vi "Detector Setup.vi"(8 "error in (no error)":errorcluster, 11 "Detector Class in":refnum<class "Detector Class.lvclass">) -> (0 "error out":errorcluster, 2 "Detector Config.Detector":u16, 3 "Detector Class out":refnum<class "Detector Class.lvclass">)   [LabVIEW 2021, in "Detector Class.lvclass"]
uses:
  Detector Class.lvclass
  Detector Class.lvclass/Detector Class.ctl
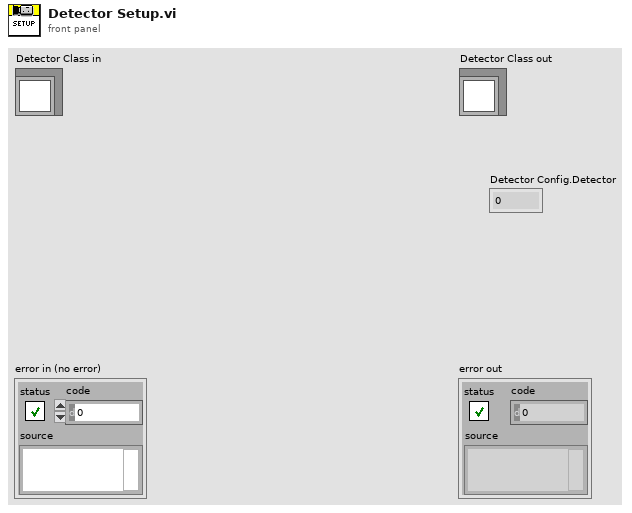
[diagram p1: front panel]
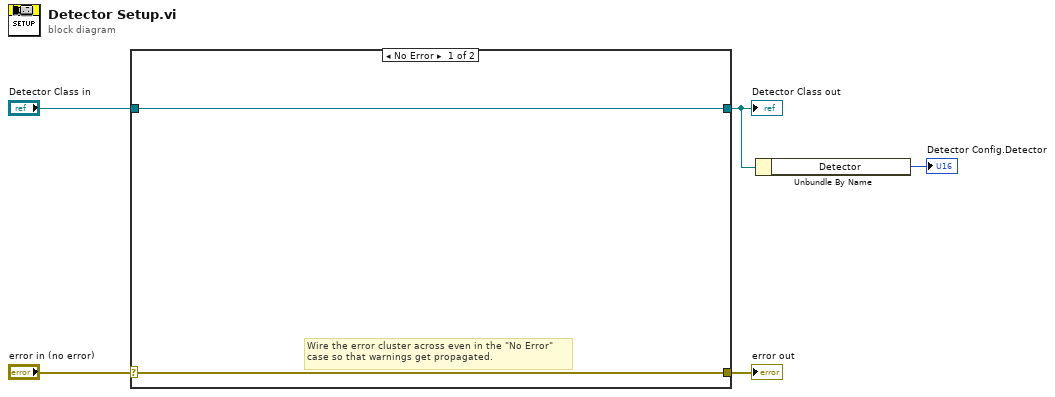
[diagram p0: block diagram]
diagram:
  n1 = case shown="No Error" "error in (no error)" {
    selector: "error in (no error)" -> [w6 w9]
    tunnel: [w6 w9] -> w4
    tunnel: [w7 w8] -> w2
    tunnel: "Detector Class in" -> [w7 w8]
    frame No Error {
      # "Wire the error cluster across even in the \"No Error\"\ncase so that warnings get propagated."
    }
    frame Error {
    }
  }
  "error out" <- w4
  "Detector Class out" <- w2
  n2 = Unbundle By Name(w2) -> ("Detector"=→"Detector Config.Detector":u16)
